vi "TEST_ASIC_SUM_(1ST).vi"(4 "Voltages comprobation":dbl[](array[numeric])=[0.05, 0.1, 0.2, 0.5, 0.8], 5 "Serial number":string="SN018", 6 "IB_Clip":i32[](array[numeric])=[7, 23, 31, 63], 7 "Save NOW!":bool, 8 "error in":errorcluster, 9 "Cycles Burst":i32=10000, 10 "Channels":i32[](array[numeric])=[0, 1, 2, 3, 4, 5, 6], 11 "Instrument VISA in":T1={"AWG VISA"="generadorpulsos", "Oscilloscope  VISA "="Oscilloscope", "Integration Board IP"="172.16.7.43", "connection ID"=refnum, "report out"=refnum, "report file path"=path "C:/Documents and Settings/CTA_LAB01/Desktop/L0_Asic/L0 Asic Test Data"}) -> (0 "error out":errorcluster, 3 "Instrument VISA out":T1={"AWG VISA"="generadorpulsos", "Oscilloscope  VISA "="Oscilloscope", "Integration Board IP"="172.16.7.43", "connection ID"=refnum, "report out"=refnum, "report file path"=path "C:/Documents and Settings/CTA_LAB01/Desktop/L0_Asic/L0 Asic Test Data"})   [LabVIEW 2012]
uses:
  <vilib>/Utility/NIReport.llb/NI_report.lvclass
  <vilib>/Utility/NIReport.llb/HTML/NI_HTML.lvclass
  <instrlib>/Agilent 8000 Series/Public/Configure/Configure Math (Binary Operation).vi
  <instrlib>/Agilent 8000 Series/Public/Data/Read (Multiple Waveforms).vi
  Sum_Abrilader/L0_Sum_Adder Folder/C/Program Files/National Instruments/LabVIEW 2012/instr.lib/Agilent 81150/Agilent 81150.lvlib
  <instrlib>/Agilent 8000 Series/Agilent 8000 Series.lvlib
panel:
  out "ClipRect":dbl=136149.0
  in  "Atenuation":i32[](array[numeric])=[0, 15]
  out "dt":dbl=3.125e-12
  out "report file path":path=path "C:/Documents and Settings/CTA_LAB01/Desktop/L0_Asic/L0 Asic Test Data"
  in  "Full waveform":bool
  out "Waveform Data":waveform(dbl)[](graph)=[{"t0"=timestamp(-6.010937525502413e-09 s since 1904-01-01), "dt"=3.125e-12, "Y"=array[6408 elements]}, {"t0"=timestamp(-6.010937525502413e-09 s since 1904-01-01), "dt"=3.125e-12, "Y"=array[6408 elements]}]
  out "time for channel bucle":u32=4294966675
  out "iindex inner bucle":u16=109
  out "time attenuation bucle":u32=136149
  out "points quantity":dbl=15.0
  out "appended array":dbl[](array[numeric])=[9.99999e+37, 9.99999e+37, 2.137332e-09, 7.2166e-11, 9.99999e+37, 9.99999e+37, 9.99999e+37, 9.99999e+37, 9.99999e+37, 9.99999e+37, 15.0]
  out "read buffer 3":string="V amptd(1),9.99999E+37,9.99999E+37,9.99999E+37,9.99999E+37,9.99999E+37,1.5E+01,+ width(1),2.18163E-09,2.01279E-09,2.26658E-09,2.137332E-09,7.2166E-11,1.5E+01,V amptd(f2),9.99999E+37,9.99999E+37,9.99999E+37,9.99999E+37,9.99999E+37,1.5E+01,+ width(f2),9.99999E+37,9.99999E+37,9.99999E+37,9.99999E+37,9.99999E+37,9E+00,Time(1-f2),9.99999E+37,9.99999E+37,9.99999E+37,9.99999E+37,9.99999E+37,1.3E+01\n"
  out "bucle for inner bucle":u32=363
  out "Numeric":i32=9300975
  in  "Clip_sel_b":u32
  in  "Att gain":u32=4095
  in  "Quantity of measurements":u32=50
  in  "End 2":bool
  out "Data output":dbl[][](array[numeric])=[[0.05, 0.0, 15.0, 7.0, 1.0, 9.99999e+37, 9.99999e+37, 2.14249e-09, 8.3497e-11, 9.99999e+37, 9.99999e+37, 9.99999e+37, 9.99999e+37, 9.99999e+37, 9.99999e+37, 17.0, 0.0336, -0.00019404761904761897, 105.0], [0.05, 0.0, 15.0, 31.0, 1.0, 9.99999e+37, 9.99999e+37, 2.188109e-09, 8.187e-11, 9.99999e+37, 9.99999e+37, 9.99999e+37, 9.99999e+37, 9.99999e+37, 9.99999e+37, 14.0, 0.0336, -0.00019404761904761897, 106.0], [0.05, 0.0, 15.0, 63.0, 1.0, 9.99999e+37, 9.99999e+37, 2.133683e-09, 8.8016e-11, 9.99999e+37, 9.99999e+37, 9.99999e+37, 9.99999e+37, 9.99999e+37, 9.99999e+37, 15.0, 0.0336, -0.00019404761904761897, 107.0], [0.05, 1.0, 15.0, 7.0, 1.0, 9.99999e+37, 9.99999e+37, 2.137332e-09, 7.2166e-11, 9.99999e+37, 9.99999e+37, 9.99999e+37, 9.99999e+37, 9.99999e+37, 9.99999e+37, 15.0, 0.0336, -0.00019404761904761897, 108.0]]
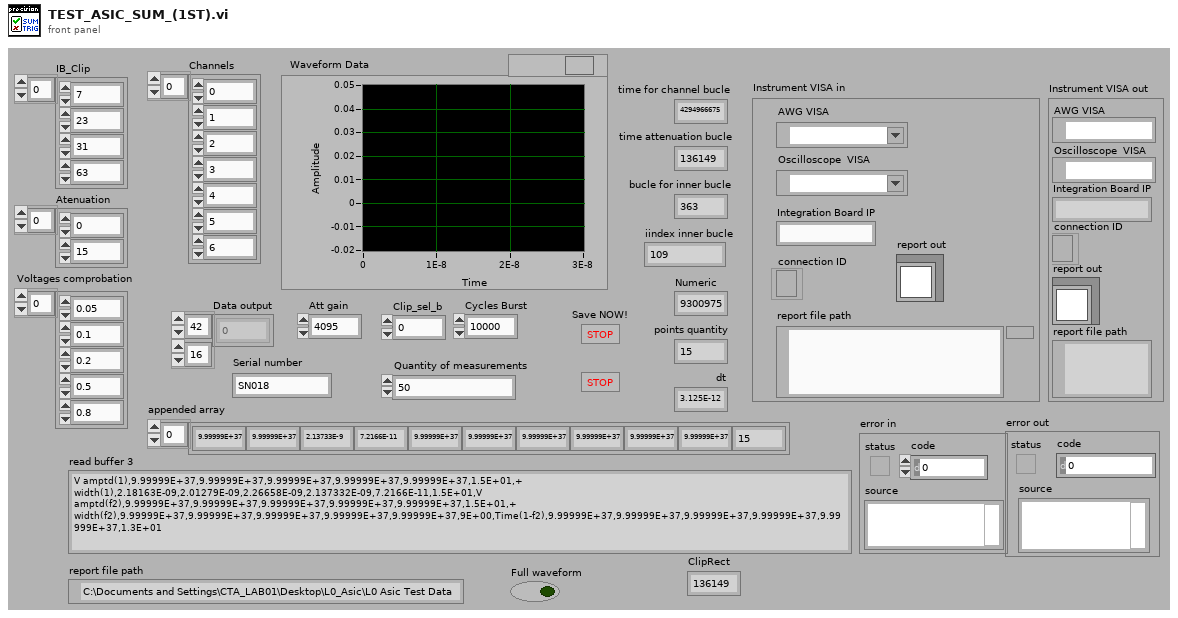
[diagram p1: front panel]
types:
  T1 = cluster{"AWG VISA":refnum<visa-resource-name>, "Oscilloscope  VISA ":refnum<visa-resource-name>, "Integration Board IP":string, "connection ID":refnum<k5>, "report out":refnum<class "NI_report.lvclass">, "report file path":path}
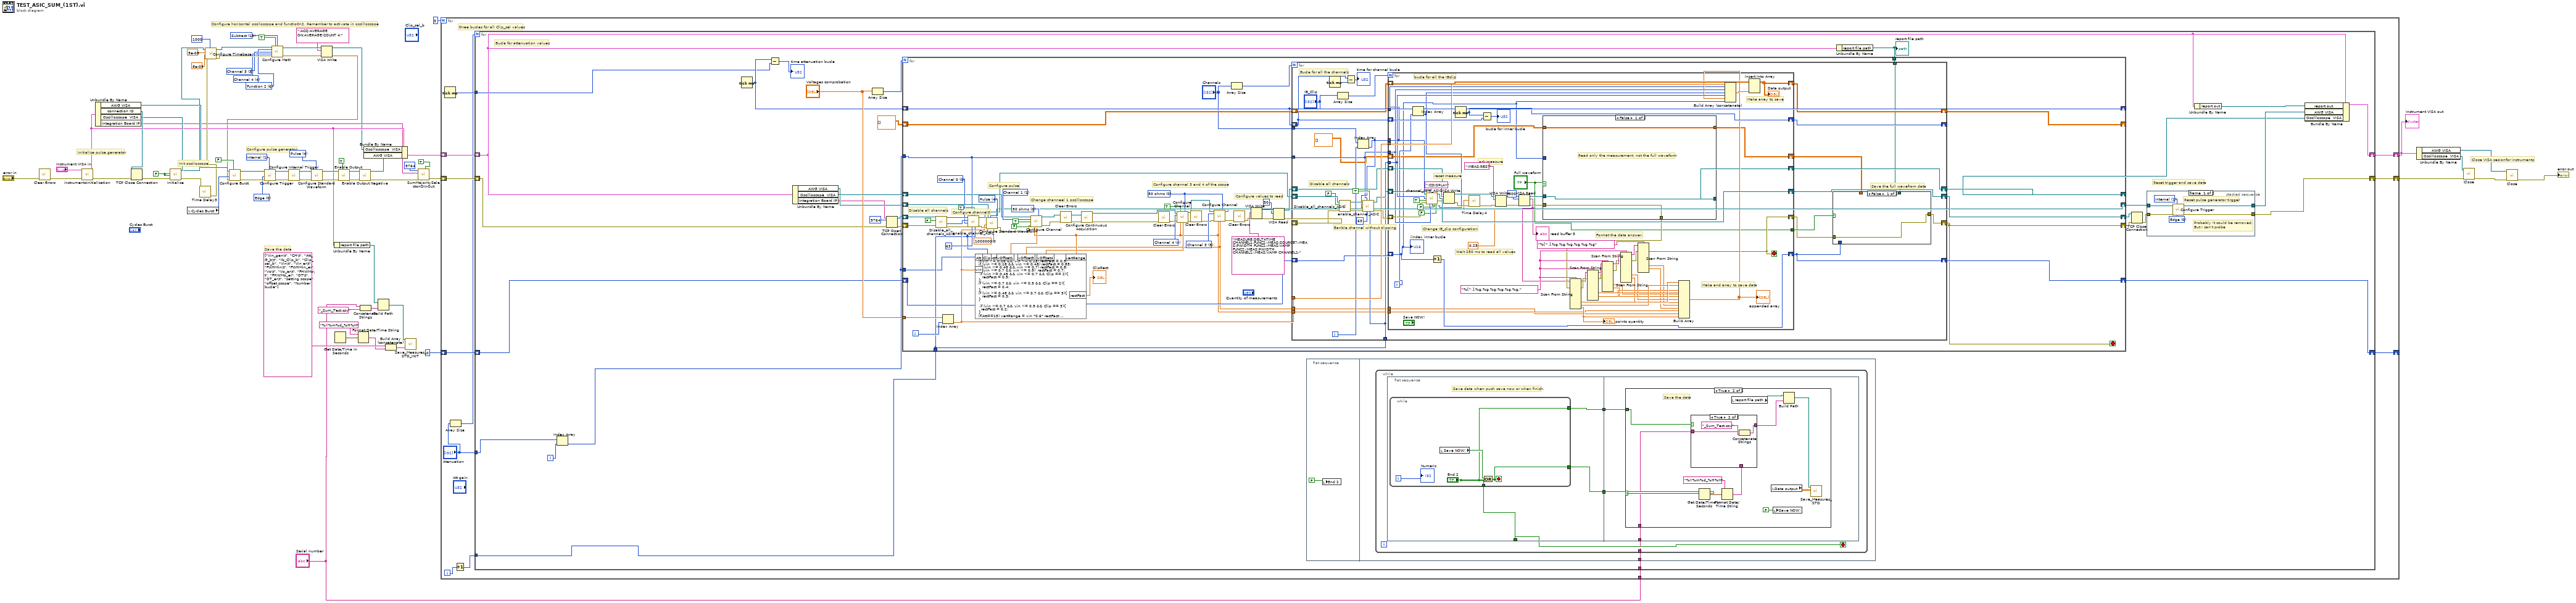
[diagram p0: block diagram]
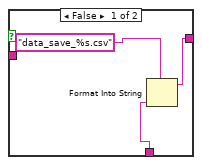
[diagram p3: hidden frame]
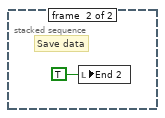
[diagram p4: hidden frame]
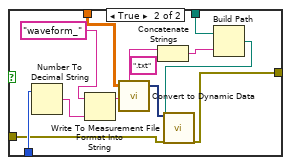
[diagram p5: hidden frame]
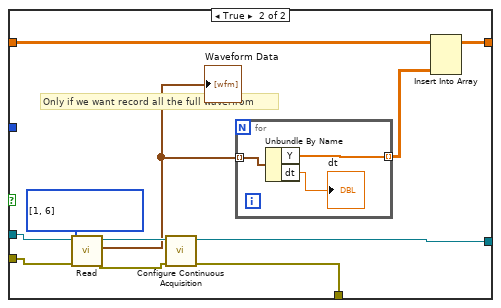
[diagram p6: hidden frame]
diagram:
  w39 = u16 6 items=["Function 1"=5, "Function 2"=6, "Function 3"=7, "Function 4"=8] ("Math Channel (5: Function 1)")
  w43 = u16 15 items=["Add"=12, "Divide"=13, "Multiply"=14, "Subtract"=15, "Common Mode"=16, "Versus"=17] ("Math Operation (12: Add)")
  w38 = 3 items=["Channel 1"=1, "Channel 2"=2, "Channel 3"=3, "Channel 4"=4] ("Channel (1: Channel 1)")
  w37 = 4 items=["Channel 1"=1, "Channel 2"=2, "Channel 3"=3, "Channel 4"=4] ("Channel (1: Channel 1)")
  w60 = u16 1 items=["Immediate", "Internal", "External", "Software Trigger Function"] ("Trigger Source (0: Immediate)")
  w61 = u16 0 items=["Edge", "Level"] ("Trigger Mode (0: Edge)")
  w65 = u16 4 items=["Sine", "Square", "Ramp Up", "Ramp Down", "Pulse", "Noise", "DC"] ("Waveform (0: Sine)")
  w69 = FALSE ("ID Query (True)")
  # "Save the data"
  # "Configure horizontal osciloscope and functio0n2. Remember to activate in oscilloscope"
  # "Close VISA sesionfor instruments"
  # "Configure pulse generator"
  # "Init osciloscope"
  # "Initialize pulse generator"
  n1 = call <vilib>:"Clear Errors.vi"("error in (no error)"="error in") -> ("error out"=w67:errorcluster)  [unwired: 6 in]
  n2 = call "instrumentsInitialization.vi"("error in"=w67, "Instrument VISA in"="Instrument VISA in") -> ("error out"=w54:errorcluster, "Instrument VISA out"=w13:T1)  [unwired: 8 in]
  n3 = Unbundle By Name(w13) -> ("AWG VISA"=w50:refnum<visa-resource-name>, "connection ID"=w55:refnum<k5>, "Oscilloscope  VISA"=w51:refnum<visa-resource-name>, "Integration Board IP"=w8:string)
  n4 = TCP Close Connection(connection ID=w55, error in (no error)=w54) -> (error out=w49:errorcluster)  [unwired: 1 in, 1 out]
  n5 = call <instrlib>:"Initialize.vi"("error in (no error)"=w49, "Reset (True)"=w69, "ID Query (True)"=w69, "VISA resource name"=w51) -> ("error out"=w68:errorcluster, "VISA resource name out"=w36:refnum<visa-resource-name>)  [unwired: 6 in]
  n6 = local read "Cycles Burst"() -> (w64:i32)
  n7 = call "Time Delay3"("error in (no error)"=w68) -> ("error out"=w35:errorcluster)  [unwired: 10 in]
  n8 = call <instrlib>:"Configure Timebase.vi"("Record Length (1000)"=1000, "error in (no error)"=w35, "Position (0.0 s)"=8e-09, "Timebase (0.005 s)"=5e-08, "VISA resource name"=w36) -> ("error out"=w40:errorcluster, "VISA resource name out"=w41:refnum<visa-resource-name>)  [unwired: 5 in]
  n9 = call-poly <instrlib>:"Configure Math.vi"("VISA resource name"=w41, "Enable Math Channel (T:Enable)"=TRUE, "Math Operation (12: Add)"=w43, "Math Channel (5: Function 1)"=w39, "Math Operand (1: Channel 1)"=w38, "Math Operand (2: Channel 2)"=w37, "error in (no error)"=w40) -> ("VISA resource name out"=w5:refnum<visa-resource-name>, "error out"=w4:errorcluster)  [unwired: 7 in]
  n10 = VISA Write(VISA resource name=w5, write buffer=":ACQ:AVERAGE ON;AVERAGE:COUNT 4;", error in (no error)=w4) -> (VISA resource name out=w2:refnum<visa-resource-name>, error out=w3:errorcluster)  [unwired: 1 out]
  n11 = call <instrlib>:"Configure Burst.vi"("Enable Burst (F: Disable)"=FALSE, "error in (no error)"=w3, "Burst Count (2)"=w64, "VISA resource name"=w50) -> ("error out"=w63:errorcluster, "VISA resource name out"=w62:refnum<visa-resource-name>)  [unwired: 6 in]
  n12 = call <instrlib>:"Configure Trigger.vi"("Trigger Source (0: Immediate)"=w60, "error in (no error)"=w63, "Trigger Mode (0: Edge)"=w61, "VISA resource name"=w62) -> ("error out"=w59:errorcluster, "VISA resource name out"=w58:refnum<visa-resource-name>)  [unwired: 6 in]
  n13 = call <instrlib>:"Configure Internal Trigger.vi"("error in (no error)"=w59, "VISA resource name"=w58) -> ("error out"=w56:errorcluster, "VISA resource name out"=w57:refnum<visa-resource-name>)  [unwired: 8 in]
  n14 = call <instrlib>:"Configure Standard Waveform.vi"("Waveform (0: Sine)"=w65, "error in (no error)"=w56, "VISA resource name"=w57) -> ("error out"=w48:errorcluster, "VISA resource name out"=w47:refnum<visa-resource-name>)  [unwired: 7 in]
  n15 = Unbundle By Name(w13) -> ("report file path"=w14:path)
  n16 = Get Date/Time In Seconds() -> (seconds since 1Jan1904=w19:timestamp)
  n17 = call <instrlib>:"Enable Output.vi"("Enable Output (T: Enable)"=TRUE, "error in (no error)"=w48, "VISA resource name"=w47) -> ("error out"=w25:errorcluster, "VISA resource name out"=w24:refnum<visa-resource-name>)  [unwired: 7 in]
  n18 = Format Date/Time String(time format string (%c)="%Y%m%d_%H%M", seconds (now)=w19) -> (date/time string=w17:string)  [unwired: 1 in]
  n19 = call "Enable Output Negative.vi"("error in (no error)"=w25, "VISA resource name"=w24) -> ("error out"=w9:errorcluster, "VISA resource name out"=w23:refnum<visa-resource-name>)  [unwired: 8 in]
  n20 = Concatenate Strings("Serial number", "_Sum_Test.csv" ("format string")) -> (w15:string)
  n21 = Bundle By Name(cluster=w13, "Oscilloscope  VISA"=w2, "AWG VISA"=w23) -> (w28:T1)
  n22 = Build Path(base path=w14, name or relative path=w15) -> (appended path=w22:path)
  n23 = Build Array (concatenate)(string[] ["Vin_gen\t", "CH\t", "Att_G_b\t", "Ib_Clip_b", "Clip_sel_b", "Vin\t", "Vin er\t", "FWHMin\t", "FWHMin_er", "Vo\t", "Vo_er\t", "FHWMo\t", "FHWMo_er", "DT\t", "DT_er\t", "setting scope", "offset scope", "Number bucle"] ("appended array"), w17) -> (w20:string[])
  n24 = call "Save_Measures_STD_INIT.vi"("appended array"=w20, "file path (dialog if empty)"=w22) -> ()  [unwired: 10 in]
  n25 = call "SumMajoritySelectorIDInOut.vi"("On Sum\nOff Majority"=TRUE ("Enable Output (T: Enable)"), "error in"=w9, "address"=w8, "remote port or service name"=u16 9764) -> ("error out"=w10:errorcluster)  [unwired: 7 in]
  n26 = for {
    N: 3 -> [_]
    shift-right: [w81] -> w30
    shift-left: w10 -> [w77]
    shift-right: [w80] -> w12
    shift-left: w28 -> [w76]
    shift-right: [w73] -> _
    shift-left: u16 0 ("remote port or service name") -> [w74]
    tunnel: "Serial number" -> [w70]
    i -> [w78]
    # "three bucles for all Clip_sel values"
    n27 = Tick Count (ms)() -> (millisecond timer value=w75:u32)
    n28 = Array Size(array="Atenuation") -> (size(s)=w72:i32)
    n29 = Increment(x=w78) -> (x+1=w79:i32)
    n30 = for {
      N: w72 -> [_]
      shift-right: [w86] -> w81
      shift-left: w77 -> [w103]
      shift-right: [w110] -> w80
      shift-left: w76 -> [w90]
      tunnel: w79 -> [w88]
      tunnel: w75 -> [w95]
      shift-right: [w93] -> w73
      shift-left: w74 -> [w94]
      tunnel: "Atenuation" -> [w84]
      tunnel: w70 -> [w83]
      i -> [w85]
      # "Reset trigger and save data"
      # "Bucle for attenuation values"
      n31 = Index Array(array=w84, index=w85) -> (element=w82:i32)
      n32 = Tick Count (ms)() -> (millisecond timer value=w96:u32)
      n33 = Subtract(x=w96, y=w95) -> (x-y=→"time attenuation bucle":u32)
      n34 = Unbundle By Name(w90) -> ("AWG VISA"=w107:refnum<visa-resource-name>, "Oscilloscope  VISA"=w108:refnum<visa-resource-name>, "Integration Board IP"=w104:string)
      n35 = Array Size(array="Voltages comprobation") -> (size(s)=w111:i32)
      n36 = TCP Open Connection(address=w104, remote port or service name=u16 9764, error in (no error)=w103) -> (connection ID=w98:refnum<k5>, error out=w102:errorcluster)  [unwired: 2 in]
      n37 = flat-sequence {
        tunnel: w83 -> [w114]
        frame #0 {
          n38 = local write "End 2"(FALSE ("End")) -> ()
        }
        frame #1 {
          n39 = while {
            tunnel: w114 -> [w115]
            stop <- w116 stop-if-true
            n40 = flat-sequence {
              tunnel: [w121] -> w118
              tunnel: [w120] -> w117
              tunnel: [w119] -> w116
              tunnel: w118 -> [w128]
              tunnel: w117 -> [w127]
              tunnel: w115 -> [w126]
              frame #0 {
                # "Save data when push save now or when finish."
                n41 = while {
                  tunnel: [w124] -> w121
                  tunnel: ["End 2"] -> w120
                  tunnel: ["End 2"] -> w119
                  i -> [w123]
                  stop <- w124 stop-if-true
                  n42 = local read "Save NOW!"() -> (w125:bool)
                  n43 = Or(x=w125, y="End 2") -> (x .or. y?=w124:bool)
                  "Numeric" <- w123
                }
              }
              frame #1 {
                n44 = case shown="True" w128 {
                  tunnel: w127 -> [_ w135]
                  tunnel: w126 -> [_ w129]
                  frame False {
                  }
                  frame True {
                    # "Save the data"
                    n45 = Get Date/Time In Seconds() -> (seconds since 1Jan1904=w132:timestamp)
                    n46 = Format Date/Time String(time format string (%c)="%Y%m%d_%H%M", seconds (now)=w132) -> (date/time string=w130:string)  [unwired: 1 in]
                    n47 = case shown="True" w135 {
                      tunnel: [w140 w142] -> w134
                      tunnel: w130 -> [w139 _]
                      tunnel: w129 -> [_ w143]
                      frame False {
                        n48 = Format Into String(format string="data_save_%s.csv", w139) -> (resulting string=w140:string)  [unwired: 2 in, 1 out]
                      }
                      frame True {
                        n49 = Concatenate Strings(w143, "_Sum_Test.csv" ("format string")) -> (w142:string)
                      }
                    }
                    n50 = local read "report file path"() -> (w133:path)
                    n51 = local read "Data output"() -> (w137:dbl[][])
                    n52 = local write "Save NOW!"(FALSE ("Save NOW!")) -> ()
                    n53 = Build Path(base path=w133, name or relative path=w134) -> (appended path=w138:path)
                    n54 = call "Save_Measures_STD.vi"("Data in"=w137, "file path (dialog if empty)"=w138) -> ()  [unwired: 10 in]
                  }
                }
              }
            }
          }
        }
      }
      n55 = Unbundle By Name(w90) -> ("report file path"=w89:path)
      "report file path" <- w89
      n56 = for {
        N: w111 -> [_]
        shift-right: [w162] -> w100
        shift-left: w102 -> [w190]
        shift-right: [w207] -> _
        shift-left: dbl[][] [] -> [w208]
        tunnel: "Voltages comprobation" -> [w206]
        shift-right: [w180] -> w109
        shift-left: w107 -> [w214]
        shift-right: [w203] -> w91
        shift-left: w108 -> [w195]
        tunnel: w82 -> [w198]
        tunnel: w88 -> [w156]
        shift-right: [w189] -> w99
        shift-left: w98 -> [w188]
        shift-right: [w165] -> _
        shift-left: w96 -> [w165]
        shift-right: [w164] -> w93
        shift-left: w94 -> [w176]
        tunnel: w89 -> [w163]
        tunnel: w82 -> [w155]
        i -> [w213]
        stop <- w162 stop-if-true
        w169 = 3 items=["Channel 1"=1, "Channel 2"=2, "Channel 3"=3, "Channel 4"=4] ("Channel (1: Channel 1)")
        w191 = 4 items=["Channel 1"=1, "Channel 2"=2, "Channel 3"=3, "Channel 4"=4] ("Channel (1: Channel 1)")
        w170 = u32 0 items=["50 ohms", "1 Mohms"] ("Input Impedance (1: 1 Mohms)")
        w197 = u16 0 items=["Channel 0", "Channel 1", "Channel 2", "Channel 3", "Channel 4", "Channel 5", "Channel 6"] ("Channel")
        w210 = u32 0 items=["50 ohms", "1 Mohms"] ("Input Impedance (1: 1 Mohms)")
        w212 = 1 items=["Channel 1"=1, "Channel 2"=2, "Channel 3"=3, "Channel 4"=4] ("Channel (1: Channel 1)")
        w215 = u16 4 items=["Sine", "Square", "Ramp Up", "Ramp Down", "Pulse", "Noise", "DC"] ("Waveform (0: Sine)")
        # "Configure values to read"
        # "Configure channel 3 and 4 of the scope"
        # "Change channeel 1 oscilloscope"
        # "Configure pulse"
        # "Configure channel0"
        # "Disable all channels"
        n57 = call "Disable_all_channels_ASIC.vi"("error in"=w190, "Clip_en_b"=FALSE, "connection ID"=w188) -> ("error out"=w201:errorcluster, "id_out"=w199:i32, "connection ID out"=w200:refnum<k5>)  [unwired: 6 in]
        n58 = Index Array(array=w206, index=w213) -> (element=w157:dbl)
        n59 = call "enable_channel_ASIC.vi"("Clip_sel_b"=w156, "maj/sum"=TRUE, "Ib_clipVb"=u32 63, "Att gain"=w198, "error in"=w201, "Channel"=w197, "id_in"=w199, "connection ID"=w200) -> ("error out"=w202:errorcluster, "connection ID out"=w182:refnum<k5>)  [unwired: 1 in, 1 out]
        n60 = formula code="float rectFact = 1;\nif(vin >= 0.08 && vin <= 0.18) rectFact = 0.9;\nif (vin >= 0.18 && vin <= 0.48) rectFact = 0.85;\n if (vin >= 0.48 && vin <= 0.7) rectFact = 0.8;\nif (vin >= 0.7 && vin <= 0.9)  rectFact = 0.7;\n if (vin >= 0.48 && vin <= 0.7 && Clip == 2){\n   rectFact = 0.5;\n}\nif (vin >= 0.7 && vin <= 0.9 && Clip == 2){\n   rectFact = 0.4;\n}\nif (vin >= 0.48 && vin <= 0.7 && Clip == 3){\n   rectFact = 0.3;\n}\n\n if (vin >= 0.7 && vin <= 0.9 && Clip == 3){\n  rectFact = 0.2;\n}\nif(Att==15) vertRange = vin *0.6* rectFact;\nelse vertRange = vin * 0.8* rectFact;\nvOffset1  = vertRange /6;\nvOffset3  = vertRange /6;\nvOffset4  = -vertRange/6;"("vin"=w157, "Att"=w155, "Clip"=w156) -> ("vOffset1"=w159:dbl, "vOffset3"=w152:dbl, "vOffset4"=w158:dbl, "vertRange"=w153:dbl, "rectFact"=→"ClipRect":dbl)
        n61 = call <instrlib>:"Configure Standard Waveform.vi"("Frequency (1000.0 Hz)"=1000000.0, "Waveform (0: Sine)"=w215, "error in (no error)"=w202, "Amplitude (1.0 Vpp)"=w157, "VISA resource name"=w214) -> ("error out"=w196:errorcluster, "VISA resource name out"=w180:refnum<visa-resource-name>)  [unwired: 5 in]
        n62 = call <instrlib>:"Configure Channel.vi"("VISA resource name"=w195, "Enable Channel (Enable)"=TRUE, "BW Limit 20MHz (Disable)"=FALSE, "Input Impedance (1: 1 Mohms)"=w210, "Channel (1: Channel 1)"=w212, "error in (no error)"=w196, "Vertical Range (2.0 V)"=w153, "Vertical Offset (0.0 V)"=w159) -> ("VISA resource name out"=w194:refnum<visa-resource-name>, "error out"=w193:errorcluster)  [unwired: 6 in]
        n63 = call <vilib>:"Clear Errors.vi"("error in (no error)"=w193) -> ("error out"=w192:errorcluster)  [unwired: 6 in]
        n64 = call <instrlib>:"Configure Continuous Acquisition.vi"("error in (no error)"=w192, "VISA resource name"=w194) -> ("error out"=w161:errorcluster, "VISA resource name out"=w160:refnum<visa-resource-name>)  [unwired: 8 in]
        n65 = call <vilib>:"Clear Errors.vi"("error in (no error)"=w161) -> ("error out"=w204:errorcluster)  [unwired: 6 in]
        n66 = call <instrlib>:"Configure Channel.vi"("VISA resource name"=w160, "Enable Channel (Enable)"=TRUE, "Input Impedance (1: 1 Mohms)"=w170, "Channel (1: Channel 1)"=w191, "error in (no error)"=w204, "Vertical Range (2.0 V)"=w153, "Vertical Offset (0.0 V)"=w158) -> ("VISA resource name out"=w172:refnum<visa-resource-name>, "error out"=w205:errorcluster)  [unwired: 7 in]
        n67 = call <vilib>:"Clear Errors.vi"("error in (no error)"=w205) -> ("error out"=w174:errorcluster)  [unwired: 6 in]
        n68 = call <instrlib>:"Configure Channel.vi"("VISA resource name"=w172, "Input Impedance (1: 1 Mohms)"=w170, "Channel (1: Channel 1)"=w169, "error in (no error)"=w174, "Vertical Range (2.0 V)"=w153, "Vertical Offset (0.0 V)"=w152) -> ("VISA resource name out"=w171:refnum<visa-resource-name>, "error out"=w175:errorcluster)  [unwired: 8 in]
        n69 = Array Size(array="Channels") -> (size(s)=w181:i32)
        n70 = call <vilib>:"Clear Errors.vi"("error in (no error)"=w175) -> ("error out"=w173:errorcluster)  [unwired: 6 in]
        n71 = VISA Write(VISA resource name=w171, write buffer="MEASURE:DELTATIME CHANNEL1,FUNC2;:MEAS:SOURCE?;:MEAS:PWIDTH FUNC2;:MEAS:VAMP FUNC2;:MEAS:PWIDTH CHANNEL1;:MEAS:VAMP CHANNEL1;", error in (no error)=w173) -> (VISA resource name out=w187:refnum<visa-resource-name>, error out=w186:errorcluster)  [unwired: 1 out]
        n72 = VISA Read(VISA resource name=w187, byte count=u32 50, error in (no error)=w186) -> (VISA resource name out=w183:refnum<visa-resource-name>, error out=w184:errorcluster)  [unwired: 2 out]
        n73 = for {
          N: w181 -> [_]
          tunnel: w198 -> [w226]
          tunnel: w156 -> [w234]
          tunnel: w157 -> [w249]
          shift-right: [w251] -> w207
          shift-left: w208 -> [w252]
          shift-right: [w250] -> w203
          shift-left: w183 -> [w247]
          shift-right: [w248] -> w189
          shift-left: w182 -> [w240]
          shift-right: [w224] -> w162
          shift-left: w184 -> [w242]
          tunnel: "Channels" -> [w246]
          shift-right: [w220] -> w164
          shift-left: w176 -> [w244]
          shift-right: [w228] -> _
          shift-left: w165 -> [w229]
          tunnel: w163 -> [w222]
          tunnel: w153 -> [w218]
          tunnel: w152 -> [w217]
          i -> [w245]
          # "Eanble channel without clipping"
          # "Disable all channels"
          # "Save the full wavefrom data"
          # "Bucle for all the channels"
          n74 = Tick Count (ms)() -> (millisecond timer value=w230:u32)
          n75 = Array Size(array="IB_Clip") -> (size(s)=w232:i32)
          n76 = call "Disable_all_channels_ASIC.vi"("error in"=w242, "Clip_en_b"=FALSE, "connection ID"=w240) -> ("error out"=w243:errorcluster, "connection ID out"=w238:refnum<k5>)  [unwired: 6 in, 1 out]
          n77 = Subtract(x=w229, y=w230) -> (x-y=→"time for channel bucle":u32)
          n78 = Index Array(array=w246, index=w245) -> (element=w235:i32)
          n79 = call "enable_channel_ASIC.vi"("Clip_sel_b"=w234, "maj/sum"=TRUE, "Ib_clipVb"=u32 63, "Att gain"=w226, "error in"=w243, "Channel"=w235, "connection ID"=w238) -> ("error out"=w241:errorcluster, "connection ID out"=w239:refnum<k5>)  [unwired: 2 in, 1 out]
          n80 = for {
            N: w232 -> [_]
            shift-right: [w275] -> w223
            shift-left: w241 -> [w299]
            tunnel: w249 -> [w330]
            shift-right: [w312] -> w251
            shift-left: w252 -> [w328]
            tunnel: w226 -> [w325]
            shift-right: [w277] -> w250
            shift-left: w247 -> [w301]
            tunnel: w234 -> [w324]
            shift-right: [w326] -> w248
            shift-left: w239 -> [w327]
            shift-right: [w321] -> w228
            shift-left: w229 -> [w322]
            tunnel: w235 -> [w284]
            shift-right: [w283] -> w220
            shift-left: w244 -> [w270]
            tunnel: "IB_Clip" -> [w282]
            shift-right: [w273] -> w221
            shift-left: dbl[][] [] ("Y") -> [w274]
            tunnel: ["Full waveform"] -> w225
            tunnel: w218 -> [w268]
            tunnel: w217 -> [w267]
            i -> [w281]
            stop <- w275 stop-if-true
            w294 = "%[^,],%g,%g,%g,%g,%g,%g," ("format string")
            # "Make and array to save data"
            # "Wait 250 ms to read all values"
            # "Change IB_clip configuration"
            # "Make array to save"
            # "Format the data answer."
            # "ask measure"
            # "reset measure"
            # "bucle for all the IBclip"
            n81 = Index Array(array=w282, index=w281) -> (element=w280:i32)
            n82 = call "channel_conf_ASIC.vi"("connection ID"=w327, "Ring"=w284, "Clip_sel_b"=w324, "CompBuf_en_b"=TRUE, "error out"=w299, "Att gain"=w325, "Ib_ClipVb"=w280, "Clip_en_b"=FALSE, "Att_en_b"=FALSE) -> ("connection ID out"=w326:refnum<k5>, "error out 2"=w297:errorcluster)  [unwired: 2 in, 3 out]
            n83 = Increment(x=w270) -> (x+1=w283:u16)
            n84 = VISA Write(VISA resource name=w301, write buffer=":CDISPLAY", error in (no error)=w297) -> (VISA resource name out=w303:refnum<visa-resource-name>, error out=w296:errorcluster)  [unwired: 1 out]
            n85 = Tick Count (ms)() -> (millisecond timer value=w321:u32)
            n86 = call "Time Delay4"("error in (no error)"=w296, "Delay Time (s)"=0.25 ("x*y")) -> ("error out"=w314:errorcluster)  [unwired: 9 in]
            n87 = Subtract(x=w321, y=w322) -> (x-y=→"bucle for inner bucle":u32)
            n88 = VISA Write(VISA resource name=w303, write buffer=":MEAS:RES?", error in (no error)=w314) -> (VISA resource name out=w319:refnum<visa-resource-name>, error out=w318:errorcluster)  [unwired: 1 out]
            n89 = VISA Read(VISA resource name=w319, byte count=u32 800, error in (no error)=w318) -> (VISA resource name out=w278:refnum<visa-resource-name>, read buffer=w315:string, error out=w279:errorcluster)  [unwired: 1 out]
            "read buffer 3" <- w315
            n90 = case shown="False" "Full waveform" {
              tunnel: w279 -> [w333 w342]
              tunnel: w278 -> [w332 w344]
              tunnel: [w332 w340] -> w277
              tunnel: [w333 w334] -> w276
              tunnel: w270 -> [_ _]
              tunnel: w274 -> [w331 w337]
              tunnel: [w331 w336] -> w273
              frame False {
                # "Read only the measurement, not the full waveform"
              }
              frame True {
                w343 = i32[] [1, 6] items=["Channel 1"=1, "Channel 2"=2, "Channel 3"=3, "Channel 4"=4, "Function 1"=5, "Function 2"=6, "Function 3"=7, "Function 4"=8, "Memory 1"=9, "Memory 2"=10, "Memory 3"=11, "Memory 4"=12] ("Channels")
                # "Only if we want record all the full waverfrom"
                n91 = call-poly <instrlib>:"Read.vi"("error in (no error)"=w342, "Channels"=w343, "VISA resource name"=w344) -> ("error out"=w339:errorcluster, "Waveform Data"=w338:waveform(dbl)[], "VISA resource name out"=w341:refnum<visa-resource-name>)  [unwired: 6 in]
                "Waveform Data" <- w338
                n92 = call <instrlib>:"Configure Continuous Acquisition.vi"("error in (no error)"=w339, "VISA resource name"=w341) -> ("error out"=w334:errorcluster, "VISA resource name out"=w340:refnum<visa-resource-name>)  [unwired: 8 in]
                n93 = for {
                  tunnel: w338 -> [w347] mode=indexing
                  tunnel: [w346] -> w335 mode=indexing
                  n94 = Unbundle By Name(w347) -> ("Y"=w346:dbl[], "dt"=→"dt":dbl)
                }
                n95 = Insert Into Array(array=w337, new element=w335) -> (w336:dbl[][])  [unwired: 2 in]
              }
            }
            n96 = Scan From String(format string=w294, input string=w315, error in=w276) -> (remaining string=w311:string, error out=w304:errorcluster, output 5=w293:dbl, output 6=w292:dbl, output 7=w269:dbl)  [unwired: 12 in, 1 out]
            "points quantity" <- w269
            n97 = Scan From String(format string=w294, input string=w311, error in=w304) -> (remaining string=w308:string, error out=w305:errorcluster, output 5=w291:dbl, output 6=w290:dbl)  [unwired: 13 in, 1 out]
            n98 = Scan From String(format string=w294, input string=w308, error in=w305) -> (remaining string=w309:string, error out=w306:errorcluster, output 5=w266:dbl, output 6=w289:dbl)  [unwired: 13 in, 1 out]
            n99 = Scan From String(format string=w294, input string=w309, error in=w306) -> (remaining string=w310:string, error out=w307:errorcluster, output 5=w288:dbl, output 6=w287:dbl)  [unwired: 13 in, 1 out]
            n100 = Scan From String(format string="%[^,],%g,%g,%g,%g,%g,%g", input string=w310, error in=w307) -> (error out=w275:errorcluster, output 5=w286:dbl, output 6=w285:dbl)  [unwired: 13 in, 2 out]
            n101 = Build Array(w293, w292, w291, w290, w266, w289, w288, w287, w286, w285, w268, w267, w269) -> (w313:dbl[])
            "appended array" <- w313
            n102 = Build Array (concatenate)(w330, w284, w325, w280, w324, w313, w270) -> (w329:dbl[])
            n103 = Insert Into Array(array=w328, new element=w329) -> (w312:dbl[][])  [unwired: 2 in]
            "Data output" <- w312
            "iindex inner bucle" <- w270
          }
          n104 = case shown="False" w225 {
            tunnel: w221 -> [_ w265]
            tunnel: w223 -> [w253 w254]
            tunnel: [w253 w263] -> w224
            tunnel: w222 -> [_ w256]
            tunnel: w220 -> [_ w255]
            frame False {
            }
            frame True {
              n105 = Number To Decimal String(number=w255) -> (decimal integer string=w262:string)  [unwired: 1 in]
              n106 = Format Into String(initial string="waveform_", w262) -> (resulting string=w260:string)  [unwired: 2 in, 1 out]
              n107 = call "Convert to Dynamic Data"("2D Array"=w265) -> ("Dynamic Data Type"=w264:dynamicdata)  [unwired: 3 in]
              n108 = Concatenate Strings(w260, ".txt" ("string")) -> (w259:string)
              n109 = Build Path(base path=w256, name or relative path=w259) -> (appended path=w257:path)
              n110 = call "Write To Measurement File"("Signals"=w264, "error in (no error)"=w254, "Filename"=w257) -> ("error out"=w263:errorcluster)  [unwired: 14 in, 2 out]
            }
          }
        }
      }
      n111 = TCP Close Connection(connection ID=w99, error in (no error)=w100) -> (error out=w101:errorcluster)  [unwired: 1 in, 1 out]
      n112 = stacked-sequence {
        tunnel: w101 -> [w148 _]
        tunnel: [w147 _] -> w86
        tunnel: w109 -> [w146 _]
        tunnel: [w145 _] -> w92
        frame #0 {
          w149 = u16 1 items=["Immediate", "Internal", "External", "Software Trigger Function"] ("Trigger Source (0: Immediate)")
          w150 = u16 0 items=["Edge", "Level"] ("Trigger Mode (0: Edge)")
          # "Probably it could be removed. \nBut I can't probe"
          # "Reset pulse generator tirgger"
          n113 = call <instrlib>:"Configure Trigger.vi"("Trigger Source (0: Immediate)"=w149, "error in (no error)"=w148, "Trigger Mode (0: Edge)"=w150, "VISA resource name"=w146) -> ("error out"=w147:errorcluster, "VISA resource name out"=w145:refnum<visa-resource-name>)  [unwired: 6 in]
        }
        frame #1 {
          # "Save data"
          n114 = local write "End 2"(TRUE ("End 2")) -> ()
        }
      }
      n115 = Unbundle By Name(w90) -> ("report out"=w87:refnum<class "NI_report.lvclass">)
      n116 = Bundle By Name(cluster=w90, "report out"=w87, "AWG VISA"=w92, "Oscilloscope  VISA"=w91) -> (w110:T1)
    }
  }
  "Instrument VISA out" <- w12
  n117 = Unbundle By Name(w12) -> ("AWG VISA"=w31:refnum<visa-resource-name>, "Oscilloscope  VISA"=w32:refnum<visa-resource-name>)
  n118 = call <instrlib>:"Close.vi"("error in (no error)"=w30, "VISA resource name"=w32) -> ("error out"=w33:errorcluster)  [unwired: 9 in]
  n119 = call <instrlib>:"Close.vi"("error in (no error)"=w33, "VISA resource name"=w31) -> ("error out"=→"error out":errorcluster)  [unwired: 9 in]
